vi "S1500_S7Com_Auswertung.vi"(8 "error in":errorcluster, 9 "Read_Data":i32[](array[numeric]), 10 "Iterationen":i32, 11 "Cluster":T1={"DB"=0, "Adresse"=0, "Länge"=0, "Typ"=enum."BYTE", "Enum"=enum."WRITE"}) -> (0 "error out":errorcluster, 1 "REAL":dbl, 2 "INT":i32, 4 "BYTE":u8, 5 "STRING":string, 6 "CHAR":string, 7 "DATA Out":string)   [LabVIEW 2018]
uses:
  S1500_ENUM Typ.ctl
  S1500_S7Com_DATATypes.ctl
  S1500_S7Com_RW.ctl
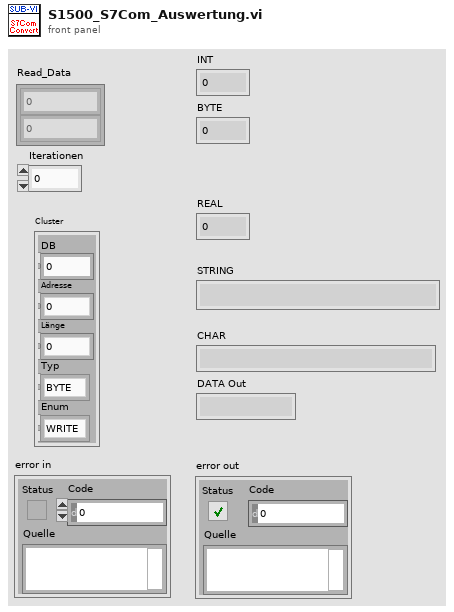
[diagram p1: front panel]
types:
  T1 = typedef "S1500_ENUM Typ.ctl" = cluster{"DB":u32, "Adresse":u32, "Länge":u32, "Typ":T2, "Enum":T3}
  T2 = typedef "S1500_S7Com_DATATypes.ctl" = enum16{"", "BIT", "BYTE", "CHAR", "WORD", "INT", "DWORD", "DINT", "REAL", "STRING"}
  T3 = typedef "S1500_S7Com_RW.ctl" = enum16{"WRITE", "READ"}
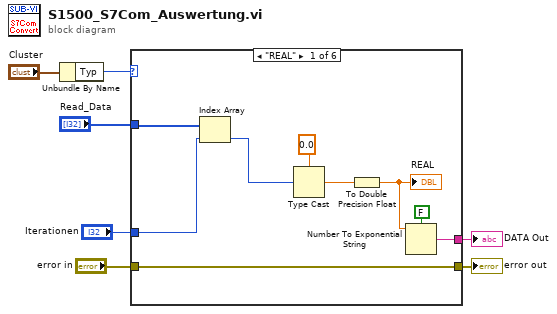
[diagram p0: block diagram]
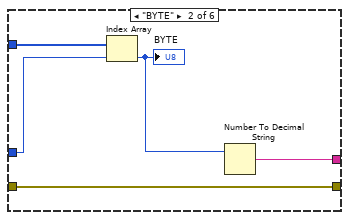
[diagram p2: hidden frame]
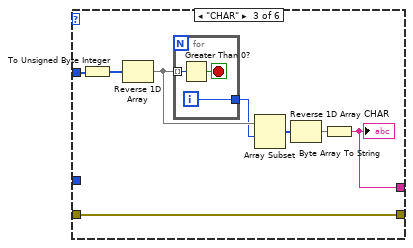
[diagram p3: hidden frame]
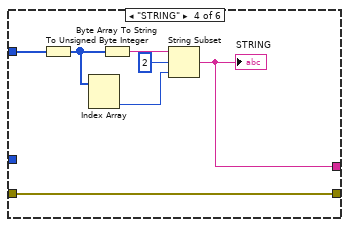
[diagram p4: hidden frame]
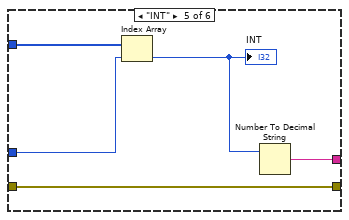
[diagram p5: hidden frame]
diagram:
  n1 = Unbundle By Name("Cluster") -> ("Typ"=w7:T2)
  n2 = case shown="\"REAL\"" w7 {
    tunnel: "Read_Data" -> [w16 w21 w29 w35 w44 _]
    tunnel: "Iterationen" -> [w15 w20 _ _ w43 _]
    tunnel: "error in" -> [w11 w19 w28 w34 w42 w45]
    tunnel: [w11 w19 w28 w34 w42 w45] -> w3
    tunnel: [w8 w17 w22 w33 w40 _] -> w2
    frame "REAL" {
      n3 = Index Array(array=w16, index=w15) -> (element=w12:i32)
      n4 = Type Cast(type=sgl 0.0, x=w12) -> (*(type *) &x=w14:sgl)
      n5 = To Double Precision Float(number=w14) -> (double precision float=w9:dbl)
      "REAL" <- w9
      n6 = Number To Exponential String(number=w9, 1:FALSE ("Systemdezimalzeichen verwenden (T)")) -> (E-format string=w8:string)  [unwired: 2 in]
    }
    frame "BYTE" {
      n7 = Index Array(array=w21, index=w20) -> (element=w18:i32)
      "BYTE" <- w18
      n8 = Number To Decimal String(number=w18) -> (decimal integer string=w17:string)  [unwired: 1 in]
    }
    frame "CHAR" {
      n9 = To Unsigned Byte Integer(number=w29) -> (unsigned 8bit integer=w23:u8[])
      n10 = Reverse 1D Array(array=w23) -> (reversed array=w27:u8[])
      n11 = for {
        tunnel: w27 -> [w32] mode=indexing
        tunnel: [w30] -> w24
        i -> [w30]
        stop <- w31 stop-if-true
        n12 = Greater Than 0?(x=w32) -> (x > 0?=w31:bool)
      }
      n13 = Array Subset(array=w27, index=w24) -> (w26:u8[])  [unwired: 1 in]
      n14 = Reverse 1D Array(array=w26) -> (reversed array=w25:u8[])
      n15 = Byte Array To String(unsigned byte array=w25) -> (string=w22:string)
      "CHAR" <- w22
    }
    frame "STRING" {
      n16 = To Unsigned Byte Integer(number=w35) -> (unsigned 8bit integer=w37:u8[])
      n17 = Index Array(array=w37) -> (element #2=w36:u8)  [unwired: 2 in, 1 out]
      n18 = Byte Array To String(unsigned byte array=w37) -> (string=w38:string)
      n19 = String Subset(string=w38, offset (0)=2 ("Offset (0)"), length (rest)=w36) -> (substring=w33:string)
      "STRING" <- w33
    }
    frame "INT" {
      n20 = Index Array(array=w44, index=w43) -> (element=w41:i32)
      "INT" <- w41
      n21 = Number To Decimal String(number=w41) -> (decimal integer string=w40:string)  [unwired: 1 in]
    }
    frame Default {
    }
  }
  "error out" <- w3
  "DATA Out" <- w2
